vi "Stop Step Trigger VI.vi"(8 "error in (no error)":errorcluster) -> (0 "error out":errorcluster)   [LabVIEW 2019, in "TimingDRV System Explorer.lvlib"]
uses:
  TimingDRV System Explorer.lvlib
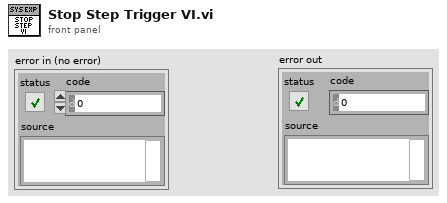
[diagram p1: front panel]
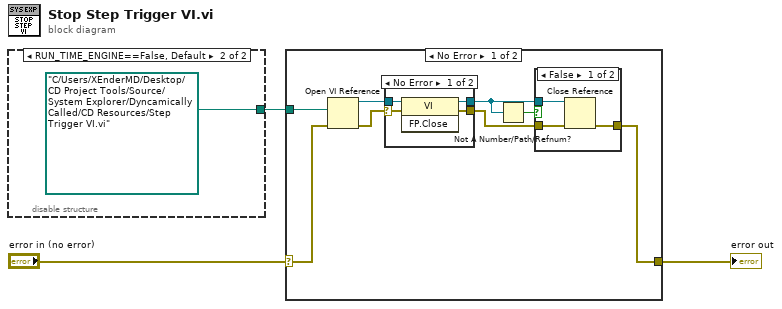
[diagram p0: block diagram]
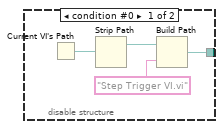
[diagram p2: hidden frame]
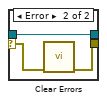
[diagram p4: hidden frame]
diagram:
  n1 = disable-structure shown="RUN_TIME_ENGINE==False, Default" {
    disable-tunnel: [w4 path "C:/Users/XEnderMD/Desktop/CD Project Tools/Source/System Explorer/Dyncamically Called/CD Resources/Step Trigger VI.vi" ("appended path")] -> w1
    frame condition #0 {
      n2 = Current VI's Path() -> (path=w7:path)
      n3 = Strip Path(path=w7) -> (stripped path=w6:path)  [unwired: 1 out]
      n4 = Build Path(base path=w6, name or relative path="Step Trigger VI.vi") -> (appended path=w4:path)
    }
    frame condition #1 (active) {
    }
  }
  n5 = case shown="No Error" "error in (no error)" {
    selector: "error in (no error)" -> [w13 w28]
    tunnel: w1 -> [w16 _]
    tunnel: [w14 w28] -> w3
    frame No Error {
      n6 = Open VI Reference(vi path=w16, error in (no error)=w13) -> (vi reference=w10:refnum<vi>, error out=w9:errorcluster)  [unwired: 4 in]
      n7 = case shown="No Error" w9 {
        selector: w9 -> [w21 w25]
        tunnel: w10 -> [w24 w26]
        tunnel: [w23 w27] -> w15
        tunnel: [w22 w26] -> w11
        frame No Error {
          n8 = invoke class="VI" method="FP.Close"(reference=w24, error in=w21) -> (reference out=w22:refnum<vi>, error out=w23:errorcluster)  [unwired: 1 in, 1 out]
        }
        frame Error {
          n9 = call <vilib>:"Clear Errors.vi"("error in (no error)"=w25) -> ("error out"=w27:errorcluster)  [unwired: 5 in, 1 out]
        }
      }
      n10 = Not A Number/Path/Refnum?(number/path/refnum=w11) -> (NaN/Path/Refnum?=w12:bool)
      n11 = case shown="False" w12 {
        tunnel: w15 -> [w19 w20]
        tunnel: [w18 w20] -> w14
        tunnel: w11 -> [w17 _]
        frame False {
          n12 = Close Reference(reference=w17, error in (no error)=w19) -> (error out=w18:errorcluster)
        }
        frame True {
        }
      }
    }
    frame Error {
    }
  }
  "error out" <- w3
